vi "Enabled.vi"(8 "error in (no error)":errorcluster, 11 "RGetSceneItemEnabled in":refnum<class "RGetSceneItemEnabled.lvclass">) -> (0 "error out":errorcluster, 2 "Enabled":bool, 3 "RGetSceneItemEnabled out":refnum<class "RGetSceneItemEnabled.lvclass">)   [LabVIEW 2020, in "obs-websocket.lvlib" / "RGetSceneItemEnabled.lvclass"]
uses:
  RGetSceneItemEnabled.lvclass
  RGetSceneItemEnabled.lvclass/RGetSceneItemEnabled.ctl
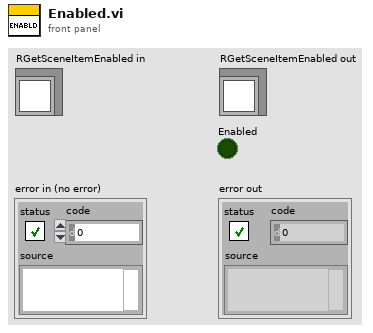
[diagram p1: front panel]
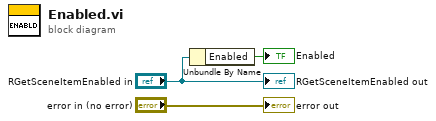
[diagram p0: block diagram]
diagram:
  n1 = Unbundle By Name("RGetSceneItemEnabled in") -> ("Enabled"=→"Enabled":bool)
  "error out" <- "error in (no error)"
  "RGetSceneItemEnabled out" <- "RGetSceneItemEnabled in"
